vi "Array2String.vi"(11 "Data_In":dbl[](array[numeric])) -> (3 "Data_out":string)   [LabVIEW 2017]
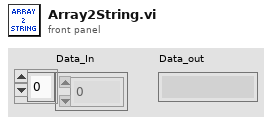
[diagram p1: front panel]
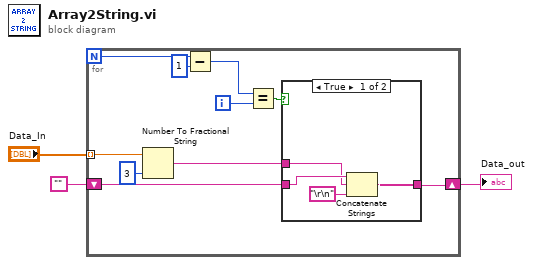
[diagram p0: block diagram]
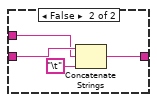
[diagram p2: hidden frame]
diagram:
  n1 = for {
    N -> [w8]
    tunnel: "Data_In" -> [w12] mode=indexing
    shift-right: [w11] -> w2
    shift-left: "" -> [w10]
    i -> [w5]
    n2 = Number To Fractional String(number=w12, precision (6)=i16 3) -> (F-format string=w9:string)  [unwired: 2 in]
    n3 = Subtract(x=w8, y=1) -> (x-y=w6:i32)
    n4 = Equal?(x=w6, y=w5) -> (x = y?=w4:bool)
    n5 = case shown="True" w4 {
      tunnel: [w17 w21] -> w11
      tunnel: w10 -> [w16 w20]
      tunnel: w9 -> [w15 w19]
      frame True {
        n6 = Concatenate Strings(w16, w15, "\r\n") -> (w17:string)
      }
      frame False {
        n7 = Concatenate Strings(w20, w19, "\t") -> (w21:string)
      }
    }
  }
  "Data_out" <- w2
